vi "close.vi"(8 "error in":errorcluster, 11 "epoll in":refnum<class "epoll.lvclass">) -> (0 "error out":errorcluster, 3 "epoll out":refnum<class "epoll.lvclass">)   [LabVIEW 2020, in "PCANBasic.lvlib" / "epoll.lvclass"]
doc: "close a file descriptor\n\nclose() closes a file descriptor, so that it no longer refers to any\n file and may be reused. Any record locks (see fcntl(2)) held on the\n file it was associated with, and owned by the process, are removed (re-\n gardless of the file descriptor that was used to obtain the lock).\n\nIf fd is the last file descriptor referring to the underlying open file\ndescription (see open(2)), the resources associated with the open file\ndescription are freed; if the descriptor was the last reference to a\nfile which has been removed using unlink(2) the file is deleted.\n\nthis vi gets executed even if there is an error upstream"
uses:
  epoll.lvclass
  epoll.lvclass/epoll.ctl
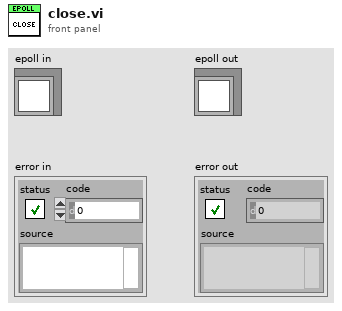
[diagram p1: front panel]
types:
  T1 = enum16{"unspecified", "close", "epoll_create", "epoll_ctl", "epoll_wait"}
  T2 = enum16{"NO ERROR", "EPERM", "ENOENT", "ESRCH", "EINTR", "EIO", "ENXIO", "E2BIG", "ENOEXEC", "EBADF", "ECHILD", "EAGAIN", "ENOMEM", "EACCES", "EFAULT", "ENOTBLK", "EBUSY", "EEXIST", "EXDEV", "ENODEV", "ENOTDIR", "EISDIR", "EINVAL", "ENFILE", "EMFILE", "ENOTTY", "ETXTBSY", "EFBIG", "ENOSPC", "ESPIPE", "EROFS", "EMLINK", "EPIPE", "EDOM", "ERANGE", "EDADLK", "ENAMETOOLONG", "ENOLCK", "ENOSYS", "ENOTEMPTY", "ELOOP", "EWOULDBLOCK", "ENOMSG", "EIDRM", "ECHRNG", "EL2NSYNC", "EL3HLT", "EL3RST", "ELNRNG", "EUNATCH", "ENOCSI", "EL2HLT", "EBADE", "EBADR", "EXFULL", "ENOANO", "EBADRQC", "EBADSLT", "EDEADLOCK", "EBFONT", "ENOSTR", "ENODATA", "ETIME", "ENOSR", "ENONET", "ENOPKG", "EREMOTE", "ENOLINK", "EADV", "ESRMNT", "ECOMM", "EPROTO", "EMULTIHOP", "EDOTDOT", "EBADMSG", "EOVERFLOW", "ENOTUNIQ", "EBADFD", "EREMCHG", "ELIBACC", "ELIBBAD", "ELIBSCN", "ELIBMAX", "ELIBEXEC", "ELISEQ", "ERESTART", "ESTRPIPE", "EUSERS", "ENOTSOCK", "EDESTADDRREQ", "EMSGSIZE", "EPROTOTYPE", "ENOPROTOOPT", "EPROTONOSUPPORT", "ESOCKTNOSUPPORT", "EOPNOTSUPP", "EPFNOSUPPORT", "EAFNOSUPPORT", "EADDRINUSE", "EADDRNOTAVAIL", "ENETDOWN", "ENETUNREACH", "ENETRESET", "ECONNABORTED", "ECONNRESET", "ENOBUFS", "EISCONN", "ENOTCONN", "ESHUTDOWN", "ETOOMANYREFS", "ETIMEDOUT", "ECONNREFUSED", "EHOSTDOWN", "EHOSTUNREACH", "EALREADY", "EINPROGRESS", "ESTALE", "EUCLEAN", "ENOTNAM", "ENAVAIL", "EISNAM", "EREMOTEIO", "EDQUOT", "ENOMEDIUM", "EMEDIUMTYPE", "ECANCELED", "ENOKEY", "EKEYEXPIRED", "EKEYREVOKED", "EKEYREJECTED", "EOWNERDEAD", "ENOTRECOVERABLE", "ERFKILL", "EHWPOISON", "UNDEFINED"}
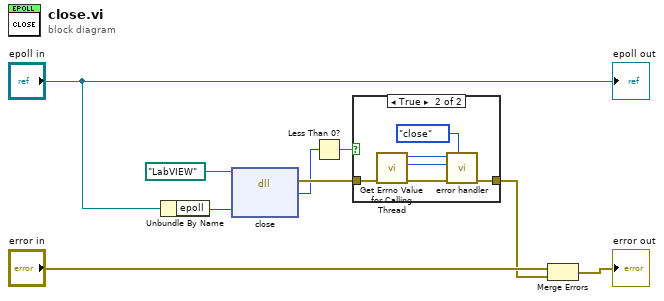
[diagram p0: block diagram]
diagram:
  n1 = Unbundle By Name("epoll in") -> ("epoll"=w6:i32)
  n2 = dll-call lib="?" fn="close"(path in=path "LabVIEW", "epoll"=w6) -> (error out=w3:errorcluster, "return"=w2:i32)  [unwired: 3 in, 1 out]
  n3 = Less Than 0?(x=w2) -> (x < 0?=w4:bool)
  n4 = case shown="True" w4 {
    tunnel: w3 -> [w10 w16]
    tunnel: [w10 w15] -> w1
    frame False {
    }
    frame True {
      n5 = call "Get Errno Value for Calling Thread.vi"("error in"=w16) -> ("error out"=w13:errorcluster, "errno number"=w12:i32, "errno"=w14:T2)  [unwired: 8 in]
      n6 = call "error handler.vi"("function (unspecified)"=T1."close", "error in"=w13, "errno number"=w12, "errno"=w14) -> ("error out"=w15:errorcluster)  [unwired: 7 in]
    }
  }
  n7 = Merge Errors("error in", w1) -> (→"error out":errorcluster)
  "epoll out" <- "epoll in"
